vi "Read Value.vi"(8 "error in (no error)":errorcluster, 11 "Bool D Element in":refnum<class "Bool D Element.lvclass">) -> (0 "error out":errorcluster, 2 "Value":bool, 3 "Bool D Element out":refnum<class "Bool D Element.lvclass">)   [LabVIEW 2018, in "D Datagrid Library.lvlib" / "Bool D Element.lvclass"]
uses:
  Bool D Element.lvclass
  Bool D Element.lvclass/Bool D Element.ctl
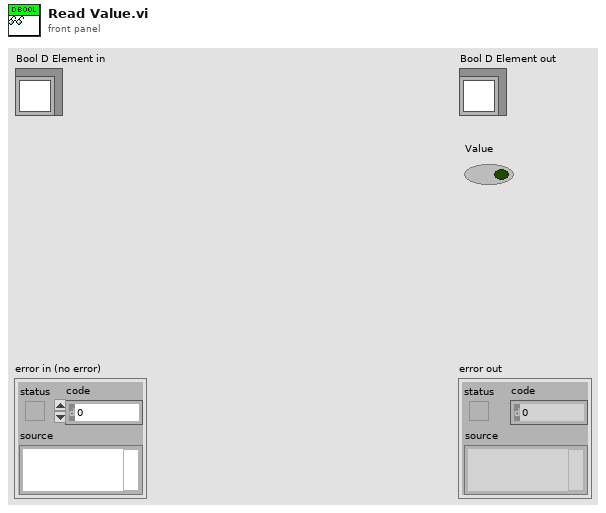
[diagram p1: front panel]
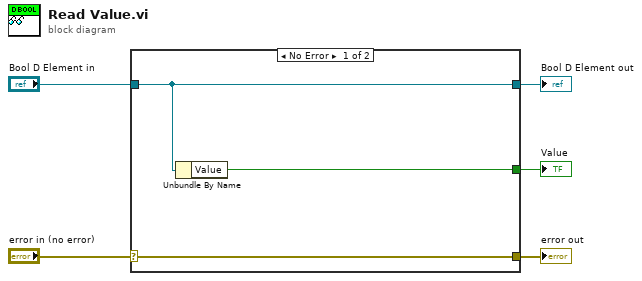
[diagram p0: block diagram]
diagram:
  n1 = case shown="No Error" "error in (no error)" {
    selector: "error in (no error)" -> [w8 w9]
    tunnel: [w8 w9] -> w4
    tunnel: [w7 w10] -> w2
    tunnel: "Bool D Element in" -> [w7 w10]
    tunnel: [w6 _] -> w1
    frame No Error {
      n2 = Unbundle By Name(w7) -> ("Value"=w6:bool)
    }
    frame Error {
    }
  }
  "error out" <- w4
  "Bool D Element out" <- w2
  "Value" <- w1
